vi "Dashboard Main.vi"() -> ()   [LabVIEW 2019]
uses:
  Corsair_V2/Team Code/TurretMode.ctl
  <vilib>/Utility/miscctls.llb/LVRowAndColumnTypeDef.ctl
  <vilib>/event_ctls.llb/eventvkey.ctl
  <vilib>/Rock Robotics/Network Tables/NT Read Boolean.vi
  <vilib>/Rock Robotics/WPI/Dashboard/WPI_DashboardLogging Global.vi
panel:
  in  "Camera Settings Right":T1={"Frame Rate"=30, "Compression"=30, "Size"=1, "DB Camera Config"=FALSE} {"Frame Rate" scale=1.0..30.0; "Compression" scale=100.0..-1.0; "Size" items=["640x480", "320x240", "160x120"]}
  in  "Camera Name Right":string(combo)="No Camera Selection"
  out "Camera Perf":string
  in  "Camera Settings":T1={"Frame Rate"=30, "Compression"=30, "Size"=1, "DB Camera Config"=FALSE} {"Frame Rate" scale=1.0..30.0; "Compression" scale=100.0..-1.0; "Size" items=["640x480", "320x240", "160x120"]}
  in  "TCP":refnum<k5>
  in  "Rec Mode":enum32{"Stop", "Record", "Playback"}(radio)
  out "Robot IP":string
  out "Image Message":string="Timeout in Camera Communications"
  in  "Dashboard Tab":T2(tab)
  in  "Autonomous Selector":u16(ring) items=["3 Ball", "5 Ball"]
  out "Intake jam?":bool
  out "Climber on?":bool
  out "Ball in conveyor?":bool
  out "A valid target?":bool
  out "Right":dbl
  out "Left":dbl
  out "Range?":bool
  out "Mode":T3(ring)=enum."Auto Disabled"
  out "Right Camera Perf":cluster{"Bandwidth (Mbps)":dbl, "FPS":dbl}
  out "Background":bool
  out "Camera Image Right":T4(plugin-control)
  out "BallState":T5(ring)
  out "TurretMode":T6
  out "ClimberState":T7(ring)
  out "RightMotorsTemperature":dbl
  out "LeftMotorsTemperature":dbl
  out "IntakeOutput":dbl
  out "RollerOutput":dbl
  out "TurretEncoder":dbl
  out "Flywheel":dbl
  in  "Select Auto":string(combo)="Select Autonomous ..."
  in  "Test Slider":dbl(slide) scale=0.0..100.0 scale format="%#_3g"
  in  "On/Off":bool caption="Solenoid"
  in  "Test Name":u16(ring) items=["Select the test to run..."]
  in  "Test Tree":string(tree)
  in  "Motor":cluster{"Value":dbl, "Enable":bool} {"Value" scale=-1.0..1.0 scale format="%#_3g"}
  out "Progress":T8 {"Test Progress" scale=0.0..100.0}
  in  "Rev/Fwd":cluster{"Forward":bool, "Reverse":bool}
  in  "Test Ring":u16(ring) items=["Monochrome", "Color"]
  out "Cmd Status":string
  in  "Execute Command":bool
  in  "Command Params":string[][](table)
  in  "Command Selection":i32(listbox)
  in  "CheckList":i32(listbox)
  out "Tree":string(tree)
  out "Camera Image":T4(plugin-control)
  in  "Camera Name":string(combo)="No Camera Selection"
  # "HW"
  # "HW"
  # "Has Limelight"
  # "Turret needs to go to:"
  # "This tab is a great place for autonomous settings and robot-specific values.\nPlace controls and indicators inside this tab and match name to\nDashboard Variables on robot. You can also delete this comment."
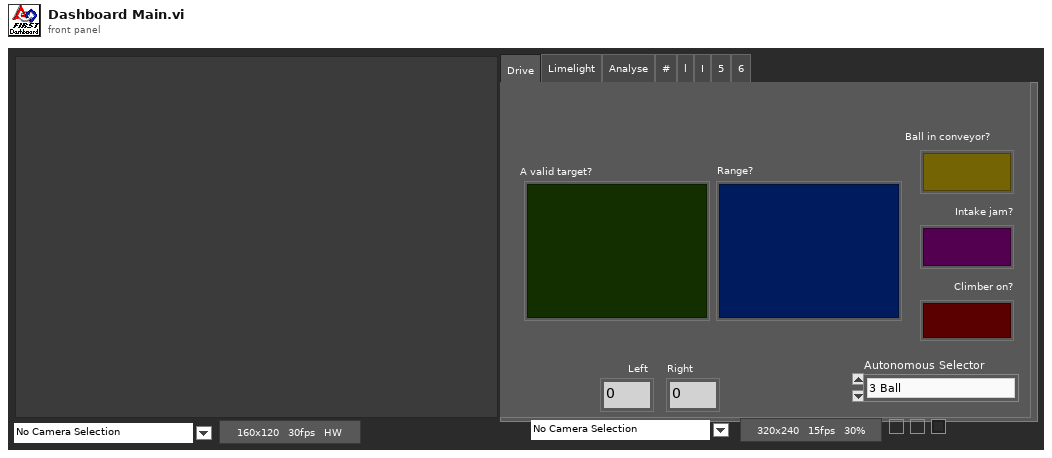
[diagram p1: front panel]
types:
  T1 = cluster{"Frame Rate":i32, "Compression":i32, "Size":u16, "DB Camera Config":bool}
  T2 = enum32{"Drive", "Limelight", "Analyse", "#", "l", "I", "5", "6"}
  T3 = enum8{"Tele-Op Disabled", "Tele-Op Enabled", "Auto Disabled", "Auto Enabled", "Test Disabled", "Test Enabled", "Disconnected", "No Code", "E-Stop"}
  T4 = typedef "IMAQ Image.ctl" = refnum<image>
  T5 = enum16{"Standart", "Get Power Cells", "Balls In", "Prepare Shooter", "Shoot!"}
  T6 = typedef "TurretMode.ctl" = enum16{"Static", "Manual", "Automatic"}
  T7 = enum16{"Standart", "Vibrate *Lenny Face*", "Open da Boi", "Engage on the Bar!", "Pull Our Hope", "Deu por Hoje"}
  T8 = cluster{"Test Progress":u8, "Test Progress Text":string}
  T9 = cluster{"Save Path":path, "Interval (s)":dbl, "Keep":i32}
  T10 = enum32{"Drive", "Camera", "Basic", "Custom", "Test", "Commands", "Checklist", "Variables"}
  T11 = typedef "Image Type" = u32
  T12 = cluster{"IDs":cluster{"RPC field ID":u16, "Unique ID":u16}, "String":string}
  T13 = cluster{"Error Strings":string, "Disable Counts":cluster{u16, u16}, "Rail Faults":cluster{u16, u16, u16}, "Robot IP":string, "DB Mode":u8, "Event Info":cluster{"Name":string, "Type":u8, "Number":u16, "Replay":u8}}
  T14 = cluster{"Storage":cluster{"Disk Free":u64, "RAM Block":u32, "RAM free":u32}, "CPU Utilization":cluster{"CPU % ISR":sgl, "CPU % Time Crit":sgl, "CPU % Timed Str":sgl, "CPU % High":sgl, "CPU % Above":sgl, "CPU % Normal":sgl, "CPU % Low":sgl}, "CAN":cluster{"% Bus Utilization":sgl, "Bus Off Cnt":u32, "TX_FIFO Full Cnt":u32, "Receive Error Cnt":u8, "Transmit Error Cnt":u8}, "HID":cluster{"HID Outputs":u32, "Rumble Low":u16, "Rumble High":u16}[]}
  T15 = cluster{"Status bits":cluster{"Test Mode":bool, "Autonomous":bool, "Enabled":bool, "Code Start":bool, "Brownout":bool, "Reserved 2":bool, "Reserved 3":bool, "E-Stop":bool}, "Code Trace":cluster{"Disabled":bool, "TeleOp":bool, "Auto":bool, "Test":bool}, "Controller Type":enum16{"unknown", "cRIO", "roboRio"}, "Code?":enum16{"unknown", "noCode", "code"}, "Battery V":dbl}
  T16 = cluster{"Control Bits":cluster{"TestMode":bool, "Autonomous":bool, "Enabled":bool, "FMS Present":bool, bool, bool, bool, "E-Stop":bool}, "Team Station ":u8, "Countdown":sgl, "Joystick Values":cluster{"Axes":dbl[], "Buttons":bool[], "POVs":i16[]}[]}
  T17 = cluster{"Camera Image":refnum<vi>, "Dashboard Tab":refnum<vi>, "Background":refnum<vi>, "Rec Mode":refnum<vi>, "Test Slider":refnum<vi>, "On/Off ":refnum<vi>, "Test Ring":refnum<vi>, "Rev/Fwd":refnum<vi>, "Test Name":refnum<vi>, "Motor":refnum<vi>, "Progress":refnum<vi>, "CheckList":refnum<vi>, "Tree":refnum<vi>, "Test Tree":refnum<vi>, "Command Params":refnum<vi>, "Command Selection":refnum<vi>, "Execute Command":refnum<vi>, "Cmd Status":refnum<vi>, "Camera Settings":refnum<vi>, "Camera Name":refnum<vi>, "Camera Perf":refnum<vi>, "Camera Settings Right":refnum<vi>, "Camera Name Right":refnum<vi>, "Camera Image Right":refnum<vi>}
  T18 = cluster{"Global Rectangle":i32[], "Contours":cluster{"Contour Type":u32, "ROI Type":u32, "Points":i32[]}[]}
  T19 = cluster{"Camera Name":string, string, "Saved DB Images Info":cluster{"Save Path":path, "Interval (s)":dbl, "Keep":i32}}
  T20 = cluster{"Camera Name Right":string, string, "Saved DB Images Info":cluster{"Save Path":path, "Interval (s)":dbl, "Keep":i32}}
  T21 = cluster{"Operation":enum16{"Update", "Clear"}, "Color Box":u32}[]
  T22 = typedef "eventvkey.ctl" = enum16{"ASCII", "Enter", "Return", "Shift", "Ctrl", "Alt", "Cmd", "Opt", "Caps", "NumLock", "Clear", "Break", "Up", "Down", "Left", "Right", "Insert", "Delete", "Home", "End", "PageUp", "PageDown", "Escape", "Help", "Pause", "ScrollLock", "F1", "F2", "F3", "F4", "F5", "F6", "F7", "F8", "F9", "F10", "F11", "F12", "F13", "F14", "F15", "F16", "F17", "F18", "F19", "F20", "F21", "F22", "F23", "F24", "Play", "VolumeUp", "VolumeDown", "Mute", "Two Byte Char"}
  T23 = cluster{"Image Size":bool, "Image Type":bool, "Pixel Value":bool, "ROI Information":bool, "Zoom Factor":bool}
  T24 = cluster{"Operation":enum16{"Update", "Clear"}, "Color Box":u32}
  T25 = typedef "LVRowAndColumnTypeDef.ctl" = cluster{"Row":i32, "Column":i32}
  T26 = cluster{"Shift":bool, "Ctrl":bool, "Alt":bool, "Cmd":bool, "Opt":bool}
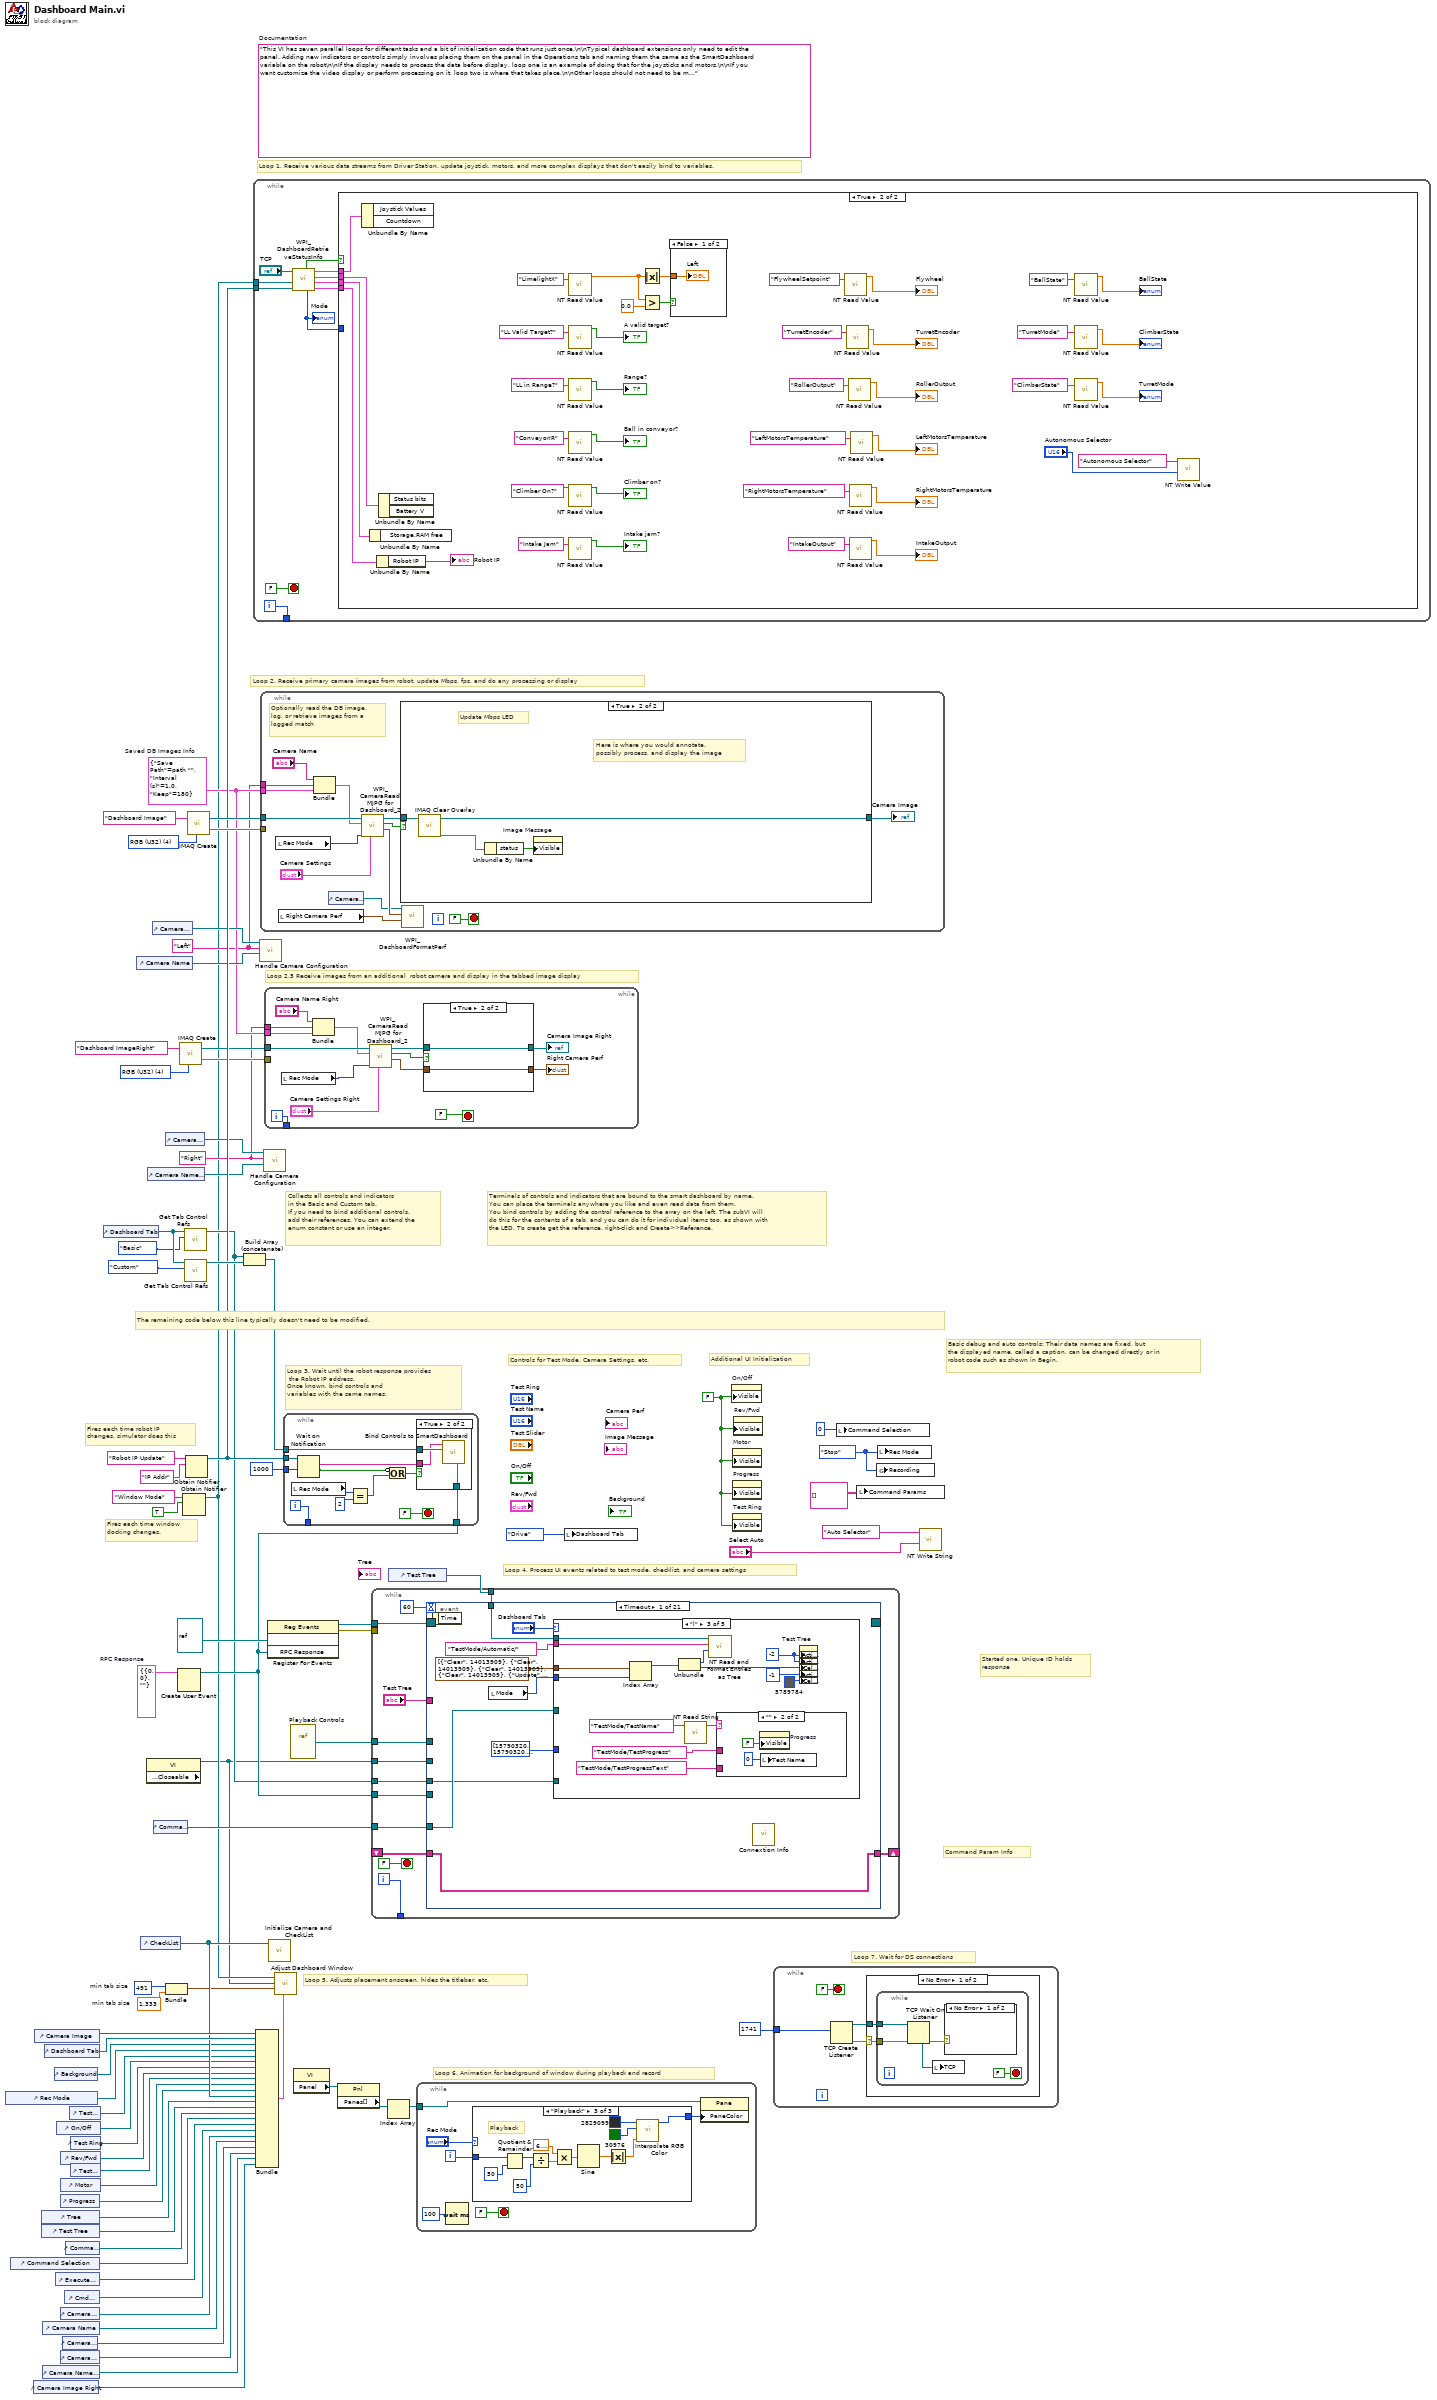
[diagram p0: block diagram]
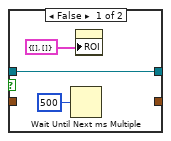
[diagram p2: hidden frame]
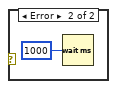
[diagram p3: hidden frame]
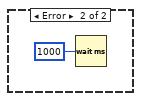
[diagram p4: hidden frame]
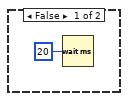
[diagram p5: hidden frame]
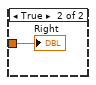
[diagram p6: hidden frame]
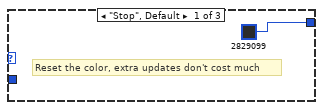
[diagram p7: hidden frame]
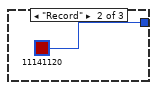
[diagram p8: hidden frame]
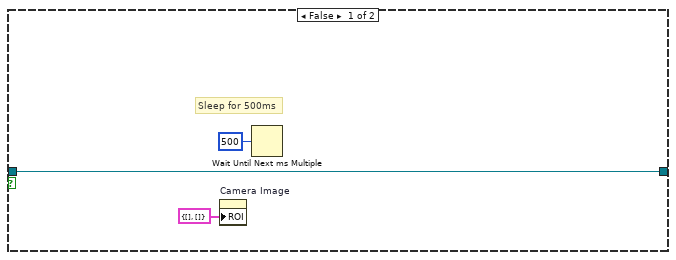
[diagram p10: hidden frame]
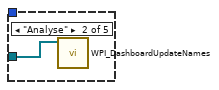
[diagram p12: hidden frame]
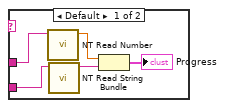
[diagram p13: hidden frame]
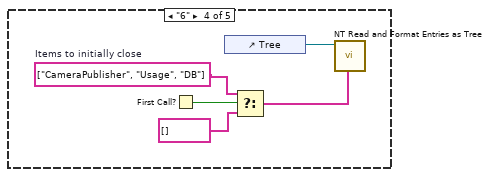
[diagram p14: hidden frame]
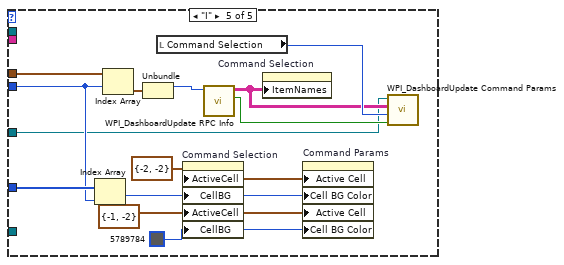
[diagram p15: hidden frame]
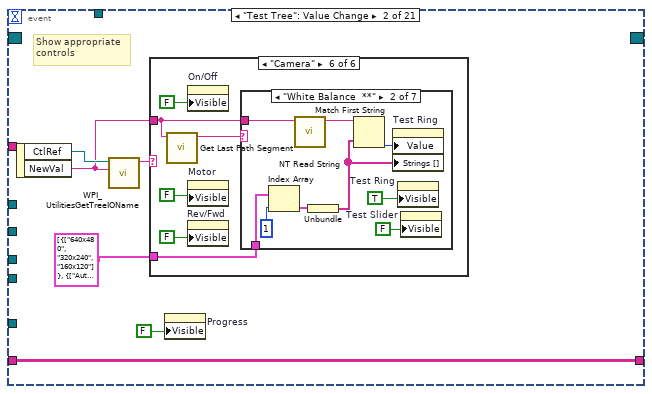
[diagram p16: hidden frame]
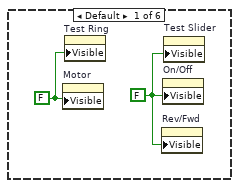
[diagram p17: hidden frame]
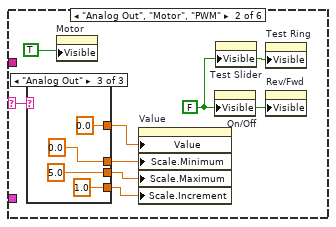
[diagram p18: hidden frame]
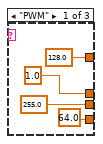
[diagram p19: hidden frame]
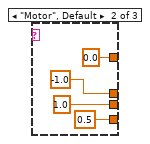
[diagram p20: hidden frame]
diagram:
  w9 = T9 {"Save Path"=path "", "Interval (s)"=1.0, "Keep"=180}  # Saved DB Images Info
  w8 = "Right"
  w7 = "Left"
  w19 = T11 4 items=["Grayscale (U8)", "Grayscale (I16)", "Grayscale (SGL)", "Complex (CSG)", "RGB (U32)", "HSL (U32)", "RGB (U64)"] ("Image Type")
  w35 = T12 {"IDs"={"RPC field ID"=0, "Unique ID"=0}, "String"=""}  # RPC Response
  w53 = 491  # min tab size
  w52 = 1.333  # min tab size
  w59 = enum32{"Stop", "Record", "Playback"}."Stop" ("Rec Mode")
  w41 = FALSE ("Visible")
  (unwired) "This VI has seven parallel loops for different tasks and a bit of initialization code that runs just once.\n\nTypical dashboard extensions only need to edit the panel. Adding new indicators or controls simply involves placing them on the panel in the Operations tab and naming them the same as the SmartDashboard variable on the robot\n\nIf the display needs to process the data before display, loop one is an example of doing that for the joysticks and motors.\n\nIf you want customize the video display or perform processing on it, loop two is where that takes place.\n\nOther loops should not need to be modified. They are pretty standard, and document the task they perform."  # Documentation
  w76 = T11 4 items=["Grayscale (U8)", "Grayscale (I16)", "Grayscale (SGL)", "Complex (CSG)", "RGB (U32)", "HSL (U32)", "RGB (U64)"] ("Image Type")
  # "Loop 2.5 Receive images from an additional  robot camera and display in the tabbed image display"
  # "Command Param Info"
  # "Started one, Unique ID holds\nresponse"
  # "Loop 7. Wait for DS connections"
  # "Basic debug and auto controls: Their data names are fixed, but\nthe displayed name, called a caption, can be changed directly or in\nrobot code such as shown in Begin."
  # "Controls for Test Mode, Camera Settings, etc."
  # "Additional UI Initialization"
  # "Loop 6. Animation for background of window during playback and record"
  # "Fires each time robot IP\nchanges, simulator does this"
  # "Fires each time window\ndocking changes."
  # "Collects all controls and indicators\nin the Basic and Custom tab.\nIf you need to bind additional controls,\nadd their references. You can extend the\nenum constant or use an integer."
  # "The remaining code below this line typically doesn't need to be modified."
  # "Loop 4. Process UI events related to test mode, checklist, and camera settings"
  # "Terminals of controls and indicators that are bound to the smart dashboard by name.\nYou can place the terminals anywhere you like and even read data from them.\nYou bind controls by adding the control reference to the array on the left. The subVI will\ndo this for the contents of a tab, and you can do it for individual items too, as shown with\nthe LED. To create get the reference, right-click and Create>>Reference."
  # "Loop 3. Wait until the robot response provides\n the Robot IP address.\nOnce known, bind controls and\nvariables with the same names."
  # "Loop 5. Adjusts placement onscreen, hides the titlebar, etc."
  # "Loop 1. Receive various data streams from Driver Station, update joystick, motors, and more complex displays that don't easily bind to variables."
  # "Loop 2. Receive primary camera images from robot, update Mbps, fps, and do any processing or display"
  n1 = control-ref of="Rec Mode"() -> (w3:refnum<vi>)
  n2 = control-ref of="Command Selection"() -> (w34:refnum<vi>)
  n3 = control-ref of="Camera Image Right"() -> (w12:refnum<vi>)
  n4 = control-ref of="Camera Image"() -> (w55:refnum<vi>)
  n5 = control-ref of="Tree"() -> (w50:refnum<vi>)
  n6 = control-ref of="Test Tree"() -> (w49:refnum<vi>)
  n7 = control-ref of="Camera Name"() -> (w25:refnum<vi>)
  n8 = control-ref of="Camera Name Right"() -> (w13:refnum<vi>)
  n9 = control-ref of="Dashboard Tab"() -> (w54:refnum<vi>)
  n10 = control-ref of="Background"() -> (w2:refnum<vi>)
  n11 = control-ref of="Execute Command"() -> (w36:refnum<vi>)
  n12 = control-ref of="On/Off"() -> (w45:refnum<vi>)
  n13 = control-ref of="Progress"() -> (w42:refnum<vi>)
  n14 = control-ref of="Camera Settings"() -> (w26:refnum<vi>)
  n15 = control-ref of="Camera Settings Right"() -> (w14:refnum<vi>)
  n16 = control-ref of="Rev/Fwd"() -> (w43:refnum<vi>)
  n17 = control-ref of="Motor"() -> (w47:refnum<vi>)
  n18 = control-ref of="Camera Perf"() -> (w24:refnum<vi>)
  n19 = control-ref of="Cmd Status"() -> (w30:refnum<vi>)
  n20 = control-ref of="Command Params"() -> (w37:refnum<vi>)
  n21 = control-ref of="Test Slider"() -> (w46:refnum<vi>)
  n22 = control-ref of="Test Ring"() -> (w44:refnum<vi>)
  n23 = control-ref of="Test Name"() -> (w48:refnum<vi>)
  n24 = control-ref of="Dashboard Tab"() -> (w58:refnum<vi>)
  n25 = control-ref of="Camera Name"() -> (w27:refnum<vi>)
  n26 = control-ref of="CheckList"() -> (w51:refnum<vi>)
  n27 = property class="VI" props=["Front Panel.Closeable"]() -> (reference out=w4:refnum<vi>)  [unwired: 2 in, 2 out]
  n28 = control-ref of="Camera Name Right"() -> (w15:refnum<vi>)
  n29 = control-ref of="Camera Settings"() -> (w28:refnum<vi>)
  n30 = control-ref of="Command Params"() -> (w29:refnum<vi>)
  n31 = control-ref of="Camera Settings Right"() -> (w16:refnum<vi>)
  n32 = Bundle("min tab size"=w53, "min tab size"=w52) -> (w6:cluster{"min tab size":i32, "min tab size":dbl})  [unwired: 1 in]
  n33 = Create User Event(user event datatype=w35) -> (user event=w31:refnum<user-event>)  [unwired: 1 in, 1 out]
  n34 = call "IMAQ Create"("Image Name"="Dashboard ImageRight", "Image Type"=w19) -> ("New Image"=w18:T4, "error out"=w17:errorcluster)  [unwired: 2 in, 1 out]
  n35 = Obtain Notifier(name (unnamed)="Window Mode", notification data type=TRUE) -> (notifier out=w5:refnum<notifier>)  [unwired: 2 in, 2 out]
  n36 = call <vilib>:"Get Tab Control Refs.vi"("Page Index"=T10."Basic" ("Dashboard Tab"), "TabControl in"=w58) -> ("ControlsOnPage"=w23:refnum<vi>[])  [unwired: 9 in]
  n37 = call <vilib>:"Get Tab Control Refs.vi"("Page Index"=T10."Custom" ("Dashboard Tab"), "TabControl in"=w58) -> ("ControlsOnPage"=w57:refnum<vi>[])  [unwired: 9 in]
  n38 = Obtain Notifier(name (unnamed)="Robot IP Update", notification data type="IP Addr" ("name (unnamed)")) -> (notifier out=w40:refnum<notifier>)  [unwired: 2 in, 2 out]
  n39 = call "IMAQ Create"("Image Name"="Dashboard Image", "Image Type"=w76) -> ("New Image"=w74:T4, "error out"=w73:errorcluster)  [unwired: 2 in, 1 out]
  n40 = Build Array (concatenate)(w23, w57) -> (w56:refnum<vi>[])
  n41 = while {
    tunnel: [w86] -> _
    tunnel: w40 -> [w80]
    tunnel: w5 -> [w77]
    i -> [w86]
    stop <- FALSE stop-if-true
    n42 = call <vilib>:"WPI_DashboardRetrieveStatusInfo.vi"("Binding Refnum"=w80, "Window Mode Notifier"=w77, "TCP Cnx"="TCP") -> ("Power and Errors"=w81:T13, "Robot Metrics"=w84:T14, "Status Info"=w85:T15, "Control Info"=w82:T16, "Robot Mode"=w79:T3, "Process?"=w83:bool)  [unwired: 3 in]
    "Mode" <- w79
    n43 = case shown="True" w83 {
      tunnel: w85 -> [_ w128]
      tunnel: w84 -> [_ w127]
      tunnel: w82 -> [_ w126]
      tunnel: w81 -> [_ w125]
      tunnel: w79 -> [_ _]
      frame False {
        n44 = Wait (ms)(milliseconds to wait=u32 20) -> ()  [unwired: 1 out]
      }
      frame True {
        n45 = Unbundle By Name(w126) -> ()  [unwired: 2 out]
        n46 = Unbundle By Name(w127) -> ()  [unwired: 1 out]
        n47 = Unbundle By Name(w125) -> ("Robot IP"=→"Robot IP":string)
        n48 = Unbundle By Name(w128) -> ()  [unwired: 2 out]
        n49 = call-poly <vilib>:"NT Read Value.vi"("Name"="LimelightX") -> ("Numeric"=w120:dbl)  [unwired: 9 in, 1 out]
        n50 = call-poly <vilib>:"NT Read Value.vi"("Name"="LL Valid Target?") -> ("Boolean"=→"A valid target?":bool)  [unwired: 9 in, 1 out]
        n51 = call-poly <vilib>:"NT Read Value.vi"("Name"="LL in Range?") -> ("Boolean"=→"Range?":bool)  [unwired: 9 in, 1 out]
        n52 = call-poly <vilib>:"NT Read Value.vi"("Name"="ConveyorIR") -> ("Boolean"=→"Ball in conveyor?":bool)  [unwired: 9 in, 1 out]
        n53 = call-poly <vilib>:"NT Read Value.vi"("Name"="Climber On?") -> ("Boolean"=→"Climber on?":bool)  [unwired: 9 in, 1 out]
        n54 = call-poly <vilib>:"NT Read Value.vi"("Name"="Intake Jam") -> ("Boolean"=→"Intake jam?":bool)  [unwired: 9 in, 1 out]
        n55 = Absolute Value(x=w120) -> (abs(x)=w119:dbl)
        n56 = Greater?(x=w120, y=0.0) -> (0:w121:bool)
        n57 = case shown="False" w121 {
          tunnel: w119 -> [w129 w130]
          frame False {
            "Left" <- w129
          }
          frame True {
            "Right" <- w130
          }
        }
        n58 = call-poly <vilib>:"NT Read Value.vi"("Name"="FlywheelSetpoint") -> ("Numeric"=→"Flywheel":dbl)  [unwired: 9 in, 1 out]
        n59 = call-poly <vilib>:"NT Read Value.vi"("Name"="TurretEncoder") -> ("Numeric"=→"TurretEncoder":dbl)  [unwired: 9 in, 1 out]
        n60 = call-poly <vilib>:"NT Read Value.vi"("Name"="RollerOutput") -> ("Numeric"=→"RollerOutput":dbl)  [unwired: 9 in, 1 out]
        n61 = call-poly <vilib>:"NT Read Value.vi"("Name"="RightMotorsTemperature") -> ("Numeric"=→"RightMotorsTemperature":dbl)  [unwired: 9 in, 1 out]
        n62 = call-poly <vilib>:"NT Read Value.vi"("Name"="IntakeOutput") -> ("Numeric"=→"IntakeOutput":dbl)  [unwired: 9 in, 1 out]
        n63 = call-poly <vilib>:"NT Read Value.vi"("Name"="LeftMotorsTemperature") -> ("Numeric"=→"LeftMotorsTemperature":dbl)  [unwired: 9 in, 1 out]
        n64 = call-poly <vilib>:"NT Read Value.vi"("Name"="BallState") -> ("Numeric"=→"BallState":dbl)  [unwired: 9 in, 1 out]
        n65 = call-poly <vilib>:"NT Read Value.vi"("Name"="TurretMode") -> ("Numeric"=→"ClimberState":dbl)  [unwired: 9 in, 1 out]
        n66 = call-poly <vilib>:"NT Read Value.vi"("Name"="ClimberState") -> ("Numeric"=→"TurretMode":dbl)  [unwired: 9 in, 1 out]
        n67 = call-poly <vilib>:"NT Write Value.vi"("Numeric"="Autonomous Selector", "Name"="Autonomous Selector") -> ()  [unwired: 9 in, 1 out]
      }
    }
  }
  n68 = Bundle("Camera Image"=w55, "Dashboard Tab"=w54, "Background"=w2, "Rec Mode"=w3, "Test Slider"=w46, "On/Off"=w45, "Test Ring"=w44, "Rev/Fwd"=w43, "Test Name"=w48, "Motor"=w47, "Progress"=w42, "CheckList"=w51, "Tree"=w50, "Test Tree"=w49, "Command Params"=w37, "Command Selection"=w34, "Execute Command"=w36, "Cmd Status"=w30, "Camera Settings"=w26, "Camera Name"=w25, "Camera Perf"=w24, "Camera Settings Right"=w14, "Camera Name Right"=w13, "Camera Image Right"=w12) -> (w1:T17)  [unwired: 1 in]
  n69 = call "Handle Camera Configuration.vi"("CameraNameRef"=w27, "Display Name"=w7, "ClusterRef"=w28) -> ()  [unwired: 9 in]
  n70 = while {
    tunnel: w74 -> [w143]
    tunnel: w73 -> [_]
    tunnel: w9 -> [w137]
    tunnel: w7 -> [w134]
    stop <- FALSE stop-if-true
    # "Optionally read the DB image,\nlog, or retrieve images from a\nlogged match"
    n71 = local read "Rec Mode"() -> (w140:enum32{"Stop", "Record", "Playback"})
    n72 = local read "Right Camera Perf"() -> (w132:cluster{"Bandwidth (Mbps)":dbl, "FPS":dbl})
    n73 = Bundle("Camera Name"="Camera Name", w134, "Saved DB Images Info"=w137) -> (w136:T19)  [unwired: 1 in]
    n74 = control-ref of="Camera Perf"() -> (w131:refnum<vi>)
    n75 = call <vilib>:"WPI_CameraRead MJPG for Dashboard_2.vi"("Camera Settings"="Camera Settings", "Rec Mode"=w140, "Capture Info"=w136, "Image in"=w143) -> ("perf info"=w133:cluster{"Bandwidth (Mbps)":dbl, "fps":dbl}, "Active"=w141:bool, "Image\\ out"=w142:T4)  [unwired: 5 in]
    n76 = case shown="True" w141 {
      tunnel: w142 -> [w146 w149]
      tunnel: [w146 w148] -> w138
      frame False {
        # "Sleep for 500ms"
        n77 = property on="Camera Image" class="ImageControl"("ROI"=T18 {"Global Rectangle"=[], "Contours"=[]}) -> ()  [unwired: 2 in, 2 out]
        n78 = Wait Until Next ms Multiple(millisecond multiple=u32 500) -> ()  [unwired: 1 out]
      }
      frame True {
        # "Here is where you would annotate,\npossibly process, and display the image"
        # "Update Mbps LED"
        n79 = call "IMAQ Clear Overlay"("Image"=w149) -> ("error out"=w150:errorcluster, "Image Out"=w148:T4)  [unwired: 2 in, 7 out]
        n80 = Unbundle By Name(w150) -> ("status"=w151:bool)
        n81 = property on="Image Message" class="Str"("Visible"=w151) -> ()  [unwired: 2 in, 2 out]
      }
    }
    "Camera Image" <- w138
    n82 = call <vilib>:"WPI_DashboardFormatPerf.vi"("Right Camera Perf"=w132, "Performance"=w133, "String in"=w131) -> ()  [unwired: 9 in]
  }
  n83 = call "Handle Camera Configuration.vi"("CameraNameRef"=w15, "Display Name"=w8, "ClusterRef"=w16) -> ()  [unwired: 9 in]
  n84 = while {
    tunnel: w18 -> [w165]
    tunnel: w17 -> [_]
    tunnel: [w160] -> _
    tunnel: w9 -> [w157]
    tunnel: w8 -> [w154]
    i -> [w160]
    stop <- FALSE stop-if-true
    n85 = local read "Rec Mode"() -> (w164:enum32{"Stop", "Record", "Playback"})
    n86 = Bundle("Camera Name Right"="Camera Name Right", w154, "Saved DB Images Info"=w157) -> (w156:T20)  [unwired: 1 in]
    n87 = call <vilib>:"WPI_CameraRead MJPG for Dashboard_2.vi"("Camera Settings"="Camera Settings Right", "Rec Mode"=w164, "Capture Info"=w156, "Image in"=w165) -> ("perf info"=w152:cluster{"Bandwidth (Mbps)":dbl, "fps":dbl}, "Active"=w159:bool, "Image\\ out"=w162:T4)  [unwired: 5 in]
    n88 = case shown="True" w159 {
      tunnel: w162 -> [w167 w170]
      tunnel: [w167 w170] -> w158
      tunnel: [_ w169] -> w153
      tunnel: w152 -> [_ w169]
      frame False {
        n89 = Wait Until Next ms Multiple(millisecond multiple=u32 500) -> ()  [unwired: 1 out]
        n90 = property on="Camera Image Right" class="ImageControl"("ROI"=T18 {"Global Rectangle"=[], "Contours"=[]}) -> ()  [unwired: 2 in, 2 out]
      }
      frame True {
      }
    }
    "Camera Image Right" <- w158
    "Right Camera Perf" <- w153
  }
  n91 = register-events(refnum<vi> refnum, w31) -> (reference out=w63:refnum<event-registration>, error out=w62:errorcluster)  [unwired: 2 in]
  n92 = call "Initialize Camera and CheckList.vi"("ListBox in"=w51) -> ()  [unwired: 11 in]
  n93 = call "Adjust Dashboard Window.vi"("Sizing Refnums"=w1, "Size Constraints"=w6, "VI"=w4, "WIn Mode"=w5) -> ()  [unwired: 8 in]
  n94 = while {
    tunnel: w56 -> [w182]
    tunnel: w40 -> [w180]
    tunnel: [w178] -> _
    tunnel: u32 1000 ("milliseconds to wait") -> [w177]
    tunnel: w31 -> [w171]
    i -> [w178]
    stop <- FALSE stop-if-true
    n95 = local read "Rec Mode"() -> (w173:enum32{"Stop", "Record", "Playback"})
    n96 = Wait on Notification(notifier=w180, timeout in ms (-1)=w177) -> (notification=w179:string, timed out?=w175:bool)  [unwired: 2 in, 2 out]
    n97 = Equal?(x=w173, y=u16 2 ("Rec Mode")) -> (x = y?=w174:bool)
    n98 = Compound Arithmetic op=OR(invert w175, w174) -> (w176:bool)
    n99 = case shown="True" w176 {
      tunnel: w182 -> [_ w185]
      tunnel: w179 -> [_ w184]
      tunnel: w171 -> [_ w183]
      frame False {
      }
      frame True {
        n100 = call <vilib>:"Bind Controls to SmartDashboard.vi"("RPC ref"=w183, "Bound Control Refs"=w185, "Server IP Address"=w184) -> ()  [unwired: 9 in]
      }
    }
  }
  n101 = vi-ref "Playback Controls.vi"() -> (w64:refnum<vi>)
  n102 = property class="VI"() -> ("Panel"=w66:refnum<vi>)  [unwired: 2 in, 2 out]
  n103 = property class="Pnl"(reference=w66) -> ("Panes[]"=w67:refnum<vi>[])  [unwired: 1 in, 2 out]
  n104 = Index Array(array=w67) -> (element=w65:refnum<vi>)  [unwired: 1 in]
  n105 = control-ref of="Test Tree"() -> (w68:refnum<vi>)
  n106 = while {
    tunnel: [w195] -> _
    tunnel: w68 -> [w194]
    tunnel: w64 -> [w193]
    tunnel: w63 -> [w192]
    tunnel: w62 -> [_]
    tunnel: w4 -> [w191]
    tunnel: w31 -> [w190]
    tunnel: w29 -> [w189]
    shift-right: [w188] -> _
    shift-left: _ -> [w187]
    tunnel: w23 -> [w186]
    i -> [w195]
    stop <- FALSE stop-if-true
    n107 = event shown="[0] Timeout" {
      selector: w192 -> [_ _ _ _ _ _ _ _ _ _ _ _ _ _ _ _ _ _ _ _ _]
      dyn-events: [_ _ _ _ _ _ _ _ _ _ _ _ _ _ _ _ w454 _ _ _ _] -> _
      timeout: u32 60 ("milliseconds to wait") -> [_ _ _ _ _ _ _ _ _ _ _ _ _ _ _ _ _ _ _ _ _]
      tunnel: w194 -> [w207 _ _ _ _ _ _ _ _ _ _ _ _ _ _ _ _ _ _ _ _]
      tunnel: "Test Tree" -> [_ _ _ _ _ _ _ _ _ _ _ w421 w429 w431 w435 w443 _ _ _ _ _]
      tunnel: w193 -> [_ _ _ _ _ _ _ _ _ _ _ _ _ _ _ _ w456 _ w474 _ _]
      tunnel: w191 -> [_ _ _ _ _ _ _ _ _ _ _ _ _ _ _ _ w452 _ _ _ _]
      tunnel: w190 -> [_ _ _ _ _ _ _ _ _ _ _ _ _ _ _ _ w450 _ _ _ _]
      tunnel: w189 -> [w203 _ _ _ _ _ w372 _ _ _ _ _ _ _ _ _ _ _ _ _ _]
      tunnel: [w202 w249 w351 w356 w365 w369 w370 w379 w389 w396 w408 w420 w427 w430 w434 w442 w449 w469 w471 w475 w488] -> w188
      tunnel: w187 -> [w202 w249 w351 w356 w365 w369 w370 _ _ w396 w408 w420 w427 w430 w434 w442 w449 w469 w471 w475 w488]
      tunnel: w186 -> [w200 _ _ _ _ _ _ _ _ _ _ _ _ _ _ _ _ _ _ _ _]
      event Timeout {
        n108 = event-data() -> ()  [unwired: 1 in, 1 out]
        n109 = local read "Mode"() -> (w205:T3)
        n110 = case shown="\"l\"" "Dashboard Tab" {
          tunnel: w207 -> [_ _ w222 _ _]
          tunnel: "TestMode/Automatic/" ("Name Pattern") -> [_ _ w221 _ _]
          tunnel: T21 [{"Operation"=enum."Clear", "Color Box"=14013909}, {"Operation"=enum."Clear", "Color Box"=14013909}, {"Operation"=enum."Clear", "Color Box"=14013909}, {"Operation"=enum."Clear", "Color Box"=14013909}, {"Operation"=enum."Update", "Color Box"=14013909}, {"Operation"=enum."Update", "Color Box"=16777215}, {"Operation"=enum."Clear", "Color Box"=14013909}, {"Operation"=enum."Clear", "Color Box"=14013909}, {"Operation"=enum."Clear", "Color Box"=14013909}] -> [_ _ w214 _ w242]
          tunnel: w205 -> [_ _ w213 _ w241]
          tunnel: u32[] [15790320, 15790320, 15790320, 15790320, 16777215, 16777215, 15790320, 15790320, 15790320] -> [_ _ _ _ w247]
          tunnel: w203 -> [_ _ _ _ w235]
          tunnel: w200 -> [_ w208 _ _ _]
          frame "Limelight", Default {
          }
          frame "Analyse" {
            n111 = call <vilib>:"WPI_DashboardUpdateNames.vi"("Controls on Tab"=w208) -> ()  [unwired: 11 in]
          }
          frame "l" {
            w220 = -2 ("Active Item:Row Number")
            n112 = Index Array(array=w214, index=w213) -> (element=w215:T24)
            n113 = Unbundle(w215) -> ("Operation"=w216:enum16{"Update", "Clear"}, "Color Box"=w217:u32)
            n114 = call <vilib>:"NT Read String.vi"("Name"="TestMode/TestName") -> ("String"=w211:string)  [unwired: 9 in, 1 out]
            n115 = call <vilib>:"NT Read and Format Entries as Tree.vi"("Operation"=w216, "Name Pattern"=w221, "Tree Refnum"=w222) -> ()  [unwired: 7 in, 2 out]
            n116 = case shown="\"\"" w211 {
              tunnel: "TestMode/TestProgress" ("Name") -> [w224 _]
              tunnel: "TestMode/TestProgressText" ("Name") -> [w223 _]
              frame Default {
                n117 = call <vilib>:"NT Read Number.vi"("Name"=w224) -> ("Numeric"=w225:dbl)  [unwired: 9 in, 1 out]
                n118 = call <vilib>:"NT Read String.vi"("Name"=w223) -> ("String"=w226:string)  [unwired: 9 in, 1 out]
                n119 = Bundle("Numeric"=w225, "String"=w226) -> (→"Progress":cluster{"Numeric":dbl, "String":string})  [unwired: 1 in]
              }
              frame "" {
                n120 = property on="Progress" class="Clust (strict)"("Visible"=FALSE) -> ()  [unwired: 2 in, 2 out]
                n121 = local write "Test Name"(u16 0) -> ()
              }
            }
            n122 = property on="Test Tree" class="Tree (strict)"("Active Item Row Number"=w220, "ActiveColNum"=w220, "CellBG"=w217, "Active Item Row Number"=-1 ("Active Item:Row Number"), "CellBG"=u32 5789784 ("Color Box")) -> ()  [unwired: 2 in, 2 out]
          }
          frame "6" {
            w232 = string[] ["CameraPublisher", "Usage", "DB"]  # Items to initially close
            n123 = First Call?() -> (First Call?: T/F=w233:bool)
            n124 = control-ref of="Tree"() -> (w234:refnum<vi>)
            n125 = Select(t=w232, s=w233, f=string[] []) -> (s? t:f=w230:string[])
            n126 = call <vilib>:"NT Read and Format Entries as Tree.vi"("Tags to  Close"=w230, "Tree Refnum"=w234) -> ()  [unwired: 8 in, 2 out]
          }
          frame "I" {
            w243 = u32 5789784 ("Color Box")
            w244 = T25 {"Row"=-1, "Column"=-2} ("Active Cell:Active Cell")
            w246 = T25 {"Row"=-2, "Column"=-2} ("Active Cell:Active Cell")
            n127 = Index Array(array=w247, index=w241) -> (element=w245:u32)
            n128 = Index Array(array=w242, index=w241) -> (element=w240:T24)
            n129 = Unbundle(w240) -> ("Operation"=w239:enum16{"Update", "Clear"})  [unwired: 1 out]
            n130 = local read "Command Selection"() -> (w238:i32)
            n131 = property on="Command Selection" class="MCListbox (strict)"("ActiveCell"=w246, "CellBG"=w245, "ActiveCell"=w244, "CellBG"=w243) -> ()  [unwired: 2 in, 2 out]
            n132 = call <vilib>:"WPI_DashboardUpdate RPC Info.vi"("Operation"=w239) -> ("update"=w237:bool, "commands"=w236:string[][])  [unwired: 9 in]
            n133 = property on="Command Selection" class="MCListbox (strict)"("ItemNames"=w236) -> ()  [unwired: 2 in, 2 out]
            n134 = property on="Command Params" class="Tbl (strict)"("Active Cell"=w246, "Cell BG Color"=w245, "Active Cell"=w244, "Cell BG Color"=w243) -> ()  [unwired: 2 in, 2 out]
            n135 = call <vilib>:"WPI_DashboardUpdate Command Params.vi"("Update"=w237, "NewVal"=w238, "Commands"=w236, "Param Tbl"=w235) -> ()  [unwired: 7 in, 1 out]
          }
        }
        n136 = call <vilib>:"Connextion Info.vi"() -> ()  [unwired: 10 in, 2 out]
      }
      event "Test Tree": Value Change {
        # "Show appropriate\ncontrols"
        n137 = event-data() -> ("CtlRef"=w252:refnum<vi>, "NewVal"=w250:string)  [unwired: 1 in]
        n138 = call <vilib>:"WPI_UtilitiesGetTreeIOName.vi"("NewVal"=w250, "TreeControl in"=w252) -> ("I/O Name"=w253:string)  [unwired: 9 in]
        n139 = case shown="\"Camera\"" w253 {
          selector: w253 -> [_ w260 _ w282 w291 _]
          tunnel: w250 -> [_ _ w279 w281 _ w298]
          tunnel: cluster{string[]}[] [{["640x480", "320x240", "160x120"]}, {["Auto", "Fixed indoor", "Fixed outdoor 1", "Fixed outdoor 2", "Fixed fluorescent 1", "Fixed fluorescent 2", "Hold current"]}, {["Auto", "Flicker-free 50 Hz", "Flicker-free 60 Hz", "Hold current"]}, {["None", "Prioritize frame rate", "Prioritize image quality"]}, {["Monochrome", "Color"]}] -> [_ _ _ _ _ w297]
          frame Default {
            w255 = FALSE ("Visible")
            w254 = FALSE ("Visible")
            n140 = property on="Motor" class="Clust (strict)"("Visible"=w254) -> ()  [unwired: 2 in, 2 out]
            n141 = property on="Test Ring" class="Ring (strict)"("Visible"=w254) -> ()  [unwired: 2 in, 2 out]
            n142 = property on="Rev/Fwd" class="Clust (strict)"("Visible"=w255) -> ()  [unwired: 2 in, 2 out]
            n143 = property on="On/Off" class="Bool (strict)"("Visible"=w255) -> ()  [unwired: 2 in, 2 out]
            n144 = property on="Test Slider" class="Slide (strict)"("Visible"=w255) -> ()  [unwired: 2 in, 2 out]
          }
          frame "Analog Out", "Motor", "PWM" {
            w261 = FALSE ("Visible")
            n145 = case shown="\"Analog Out\"" w260 {
              tunnel: [1.0 ("Value") -1.0 ("Value") 0.0 ("Value")] -> w259
              tunnel: [255.0 ("Value") 1.0 ("Value") 5.0 ("Value")] -> w258
              tunnel: [128.0 ("Value") 0.0 ("Value") 0.0 ("Value")] -> w257
              tunnel: [64.0 ("Value") 0.5 ("Value") 1.0 ("Value")] -> w256
              frame "PWM" {
              }
              frame "Motor", Default {
              }
              frame "Analog Out" {
              }
            }
            n146 = property on="Motor" class="Clust (strict)"("Visible"=TRUE) -> ()  [unwired: 2 in, 2 out]
            n147 = property on="Value" class="Slide (strict)"("Value"=w257, "Scale.Minimum"=w259, "Scale.Maximum"=w258, "Scale.Increment"=w256) -> ()  [unwired: 2 in, 2 out]
            n148 = property on="On/Off" class="Bool (strict)"("Visible"=w261) -> ()  [unwired: 2 in, 2 out]
            n149 = property on="Test Slider" class="Slide (strict)"("Visible"=w261) -> ()  [unwired: 2 in, 2 out]
            n150 = property on="Test Ring" class="Ring (strict)"("Visible"=w261) -> ()  [unwired: 2 in, 2 out]
            n151 = property on="Rev/Fwd" class="Clust (strict)"("Visible"=w261) -> ()  [unwired: 2 in, 2 out]
          }
          frame "Servo" {
            w277 = FALSE ("Visible")
            n152 = call <vilib>:"NT Read Number.vi"("Name"=w279) -> ("Numeric"=w278:dbl)  [unwired: 9 in, 1 out]
            n153 = property on="Test Slider" class="Slide (strict)"("Visible"=TRUE, "Scale.Maximum"=170.0 ("Scale.Range:Maximum")) -> ()  [unwired: 2 in, 2 out]
            n154 = local write "Test Slider"(w278) -> ()
            n155 = property on="Motor" class="Clust (strict)"("Visible"=w277) -> ()  [unwired: 2 in, 2 out]
            n156 = property on="Rev/Fwd" class="Clust (strict)"("Visible"=w277) -> ()  [unwired: 2 in, 2 out]
            n157 = property on="On/Off" class="Bool (strict)"("Visible"=w277) -> ()  [unwired: 2 in, 2 out]
            n158 = property on="Test Ring" class="Ring (strict)"("Visible"=w277) -> ()  [unwired: 2 in, 2 out]
          }
          frame "Relay", "Solenoid" {
            w280 = FALSE ("Visible")
            n159 = property on="Motor" class="Clust (strict)"("Visible"=w280) -> ()  [unwired: 2 in, 2 out]
            n160 = property on="Test Slider" class="Slide (strict)"("Visible"=w280) -> ()  [unwired: 2 in, 2 out]
            n161 = Search and Replace String(input string=w281, search string="/Value  **", replace string="/Direction") -> (result string=w287:string)  [unwired: 5 in, 3 out]
            n162 = property on="Test Ring" class="Ring (strict)"("Visible"=w280) -> ()  [unwired: 2 in, 2 out]
            n163 = call <vilib>:"NT Read String.vi"("Name"=w287) -> ("String"=w285:string)  [unwired: 9 in, 1 out]
            n164 = Equal?(x="Both directions", y=w285) -> (x = y?=w283:bool)
            n165 = Not(x=w283) -> (.not. x?=w284:bool)
            n166 = property on="Rev/Fwd" class="Clust (strict)"("Visible"=w283) -> ()  [unwired: 2 in, 2 out]
            n167 = property on="On/Off" class="Bool (strict)"("Visible"=w284, "Caption.Text"=w282) -> ()  [unwired: 2 in, 2 out]
          }
          frame "Compressor", "Digital Out" {
            w290 = FALSE ("Visible")
            # "Get direction and finish"
            n168 = property on="Motor" class="Clust (strict)"("Visible"=w290) -> ()  [unwired: 2 in, 2 out]
            n169 = property on="Test Slider" class="Slide (strict)"("Visible"=w290) -> ()  [unwired: 2 in, 2 out]
            n170 = property on="Test Ring" class="Ring (strict)"("Visible"=w290) -> ()  [unwired: 2 in, 2 out]
            n171 = property on="On/Off" class="Bool (strict)"("Visible"=TRUE, "Caption.Text"=w291) -> ()  [unwired: 2 in, 2 out]
            n172 = property on="Rev/Fwd" class="Clust (strict)"("Visible"=FALSE) -> ()  [unwired: 2 in, 2 out]
          }
          frame "Camera" {
            n173 = call <vilib>:"Get Last Path Segment.vi"("String in"=w298) -> ("String out"=w299:string)  [unwired: 10 in]
            n174 = property on="On/Off" class="Bool (strict)"("Visible"=FALSE) -> ()  [unwired: 2 in, 2 out]
            n175 = property on="Motor" class="Clust (strict)"("Visible"=FALSE) -> ()  [unwired: 2 in, 2 out]
            n176 = property on="Rev/Fwd" class="Clust (strict)"("Visible"=FALSE) -> ()  [unwired: 2 in, 2 out]
            n177 = case shown="\"White Balance  **\"" w299 {
              tunnel: w298 -> [w305 w314 w323 w332 w341 _ w347]
              tunnel: w297 -> [w303 w311 w320 w329 w338 _ _]
              frame "Size  **" {
                n178 = Index Array(array=w303) -> (element=w302:cluster{string[]})  [unwired: 1 in]
                n179 = call <vilib>:"NT Read String.vi"("Name"=w305) -> ("String"=w304:string)  [unwired: 9 in, 1 out]
                n180 = Unbundle(w302) -> (w300:string[])
                n181 = Match First String(2:w300, 3:w304) -> (0:w301:i32)  [unwired: 1 out]
                n182 = property on="Test Ring" class="Ring (strict)"("Value"=w301, "Strings []"=w300) -> ()  [unwired: 2 in, 2 out]
                n183 = property on="Test Ring" class="Ring (strict)"("Visible"=TRUE) -> ()  [unwired: 2 in, 2 out]
                n184 = property on="Test Slider" class="Slide (strict)"("Visible"=FALSE) -> ()  [unwired: 2 in, 2 out]
              }
              frame "White Balance  **" {
                n185 = Index Array(array=w311, index=1) -> (element=w312:cluster{string[]})
                n186 = call <vilib>:"NT Read String.vi"("Name"=w314) -> ("String"=w313:string)  [unwired: 9 in, 1 out]
                n187 = Unbundle(w312) -> (w309:string[])
                n188 = Match First String(2:w309, 3:w313) -> (0:w308:i32)  [unwired: 1 out]
                n189 = property on="Test Ring" class="Ring (strict)"("Value"=w308, "Strings []"=w309) -> ()  [unwired: 2 in, 2 out]
                n190 = property on="Test Ring" class="Ring (strict)"("Visible"=TRUE) -> ()  [unwired: 2 in, 2 out]
                n191 = property on="Test Slider" class="Slide (strict)"("Visible"=FALSE) -> ()  [unwired: 2 in, 2 out]
              }
              frame "Exposure  **" {
                n192 = Index Array(array=w320, index=2) -> (element=w321:cluster{string[]})
                n193 = call <vilib>:"NT Read String.vi"("Name"=w323) -> ("String"=w322:string)  [unwired: 9 in, 1 out]
                n194 = Unbundle(w321) -> (w317:string[])
                n195 = Match First String(2:w317, 3:w322) -> (0:w318:i32)  [unwired: 1 out]
                n196 = property on="Test Ring" class="Ring (strict)"("Value"=w318, "Strings []"=w317) -> ()  [unwired: 2 in, 2 out]
                n197 = property on="Test Ring" class="Ring (strict)"("Visible"=TRUE) -> ()  [unwired: 2 in, 2 out]
                n198 = property on="Test Slider" class="Slide (strict)"("Visible"=FALSE) -> ()  [unwired: 2 in, 2 out]
              }
              frame "Exposure Priority  **" {
                n199 = Index Array(array=w329, index=3) -> (element=w330:cluster{string[]})
                n200 = call <vilib>:"NT Read String.vi"("Name"=w332) -> ("String"=w331:string)  [unwired: 9 in, 1 out]
                n201 = Unbundle(w330) -> (w326:string[])
                n202 = Match First String(2:w326, 3:w331) -> (0:w327:i32)  [unwired: 1 out]
                n203 = property on="Test Ring" class="Ring (strict)"("Value"=w327, "Strings []"=w326) -> ()  [unwired: 2 in, 2 out]
                n204 = property on="Test Ring" class="Ring (strict)"("Visible"=TRUE) -> ()  [unwired: 2 in, 2 out]
                n205 = property on="Test Slider" class="Slide (strict)"("Visible"=FALSE) -> ()  [unwired: 2 in, 2 out]
              }
              frame "Color Enable  **" {
                n206 = Index Array(array=w338, index=4) -> (element=w339:cluster{string[]})
                n207 = call <vilib>:"NT Read String.vi"("Name"=w341) -> ("String"=w340:string)  [unwired: 9 in, 1 out]
                n208 = Unbundle(w339) -> (w335:string[])
                n209 = Match First String(2:w335, 3:w340) -> (0:w336:i32)  [unwired: 1 out]
                n210 = property on="Test Ring" class="Ring (strict)"("Value"=w336, "Strings []"=w335) -> ()  [unwired: 2 in, 2 out]
                n211 = property on="Test Ring" class="Ring (strict)"("Visible"=TRUE) -> ()  [unwired: 2 in, 2 out]
                n212 = property on="Test Slider" class="Slide (strict)"("Visible"=FALSE) -> ()  [unwired: 2 in, 2 out]
              }
              frame Default {
                n213 = property on="Test Ring" class="Ring (strict)"("Visible"=FALSE) -> ()  [unwired: 2 in, 2 out]
                n214 = property on="Test Slider" class="Slide (strict)"("Visible"=FALSE) -> ()  [unwired: 2 in, 2 out]
              }
              frame "Brightness  **", "Color Level  **", "Compression  **", "FPS  **", "Sharpness  **" {
                n215 = call <vilib>:"NT Read Number.vi"("Name"=w347) -> ("Numeric"=w346:dbl)  [unwired: 9 in, 1 out]
                n216 = local write "Test Slider"(w346) -> ()
                n217 = property on="Test Slider" class="Slide (strict)"("Visible"=TRUE, "Scale.Maximum"=100.0 ("Scale.Range:Maximum")) -> ()  [unwired: 2 in, 2 out]
                n218 = property on="Test Ring" class="Ring (strict)"("Visible"=FALSE) -> ()  [unwired: 2 in, 2 out]
              }
            }
          }
        }
        n219 = property on="Progress" class="Clust (strict)"("Visible"=FALSE) -> ()  [unwired: 2 in, 2 out]
      }
      event "Test Name": Mouse Enter {
        # "Populate the ring with the list of tests"
        n220 = event-data() -> ()  [unwired: 1 in, 1 out]
        n221 = call <vilib>:"NT Read String Array.vi"("Name"="TestMode/TestList") -> ("String Array"=w355:string[])  [unwired: 9 in, 1 out]
        n222 = Build Array (concatenate)("Select the test to run...", w355) -> (w354:string[])
        n223 = property on="Test Name" class="Ring (strict)"("Strings []"=w354) -> ()  [unwired: 2 in, 2 out]
      }
      event "Test Name": Value Change {
        w357 = FALSE ("Visible")
        # "Tell the robot the test name to run"
        n224 = event-data() -> ("NewVal"=w361:u16)  [unwired: 1 in]
        n225 = property on="Test Name" class="Ring (strict)"() -> ("Strings []"=w362:string[])  [unwired: 2 in, 2 out]
        n226 = local write "Progress"(T8 {"Test Progress"=0, "Test Progress Text"=""} ("Progress")) -> ()
        n227 = Index Array(array=w362, index=w361) -> (element=w360:string)
        n228 = call <vilib>:"NT Write String.vi"("String"=w360, "Name"="TestMode/TestName") -> ()  [unwired: 9 in, 1 out]
        n229 = property on="Progress" class="Clust (strict)"("Visible"=TRUE) -> ()  [unwired: 2 in, 2 out]
        n230 = property on="Motor" class="Clust (strict)"("Visible"=w357) -> ()  [unwired: 2 in, 2 out]
        n231 = property on="Test Slider" class="Slide (strict)"("Visible"=w357) -> ()  [unwired: 2 in, 2 out]
        n232 = property on="On/Off" class="Bool (strict)"("Visible"=w357) -> ()  [unwired: 2 in, 2 out]
        n233 = property on="Rev/Fwd" class="Clust (strict)"("Visible"=w357) -> ()  [unwired: 2 in, 2 out]
        n234 = property on="Test Ring" class="Ring (strict)"("Visible"=w357) -> ()  [unwired: 2 in, 2 out]
      }
      event "Select Auto": Mouse Enter {
        # "Populate the combo box with the list of autonomous options"
        n235 = event-data() -> ()  [unwired: 1 in, 1 out]
        n236 = call <vilib>:"NT Read String Array.vi"("Name"="Auto List") -> ("String Array"=w364:string[])  [unwired: 9 in, 1 out]
        n237 = property on="Select Auto" class="CmbBox"("Strings[]"=w364) -> ()  [unwired: 2 in, 2 out]
      }
      event "Select Auto": Value Change {
        # "User modified the Auto Selection. Write to NT variable so robot knows."
        n238 = event-data() -> ("NewVal"=w367:string)  [unwired: 1 in]
        n239 = call <vilib>:"NT Write String.vi"("String"=w367, "Name"="Auto Selector") -> ()  [unwired: 9 in, 1 out]
      }
      event "Command Selection": Value Change {
        # "Get the params and show in table"
        n240 = event-data() -> ("NewVal"=w373:i32)  [unwired: 1 in]
        n241 = property on="Command Selection" class="MCListbox (strict)"() -> ("ItemNames"=w371:string[][])  [unwired: 2 in, 2 out]
        n242 = call <vilib>:"WPI_DashboardUpdate Command Params.vi"("NewVal"=w373, "Commands"=w371, "Param Tbl"=w372) -> ()  [unwired: 8 in, 1 out]
      }
      event "Execute Command": Value Change {
        # "Started one, Unique ID holds\nresponse"
        n243 = event-data() -> ()  [unwired: 1 in, 1 out]
        n244 = property on="Command Selection" class="MCListbox (strict)"() -> ("ItemNames"=w384:string[][])  [unwired: 2 in, 2 out]
        n245 = Index Array(array=w384, index (row)="Command Selection", index (col)=0) -> (element=w382:string)
        n246 = call <vilib>:"Invoke Commands.vi"("Command Params"="Command Params", "Function Name"=w382) -> ("Params"=w378:u8, "Started"=w377:bool)  [unwired: 7 in, 1 out]
        n247 = Array Subset(array="Command Params", length (row)=w378) -> (w379:string[][])  [unwired: 3 in]
        n248 = Select(t="Executing" ("Cmd Status"), s=w377, f="" ("Cmd Status")) -> (s? t:f=→"Cmd Status":string)
      }
      event "Command Selection": Double Click {
        n249 = event-data() -> ("Row"=w392:i32)  [unwired: 1 in]
        n250 = property on="Command Selection" class="MCListbox (strict)"() -> ("ItemNames"=w395:string[][])  [unwired: 2 in, 2 out]
        n251 = local read "Command Params"() -> (w391:string[][])
        n252 = Index Array(array=w395, index (row)=w392, index (col)=0) -> (element=w393:string)
        n253 = call <vilib>:"Invoke Commands.vi"("Command Params"=w391, "Function Name"=w393) -> ("Params"=w390:u8, "Started"=w385:bool)  [unwired: 7 in, 1 out]
        n254 = Array Subset(array=w391, length (row)=w390) -> (w389:string[][])  [unwired: 3 in]
        n255 = Select(t="Executing" ("Cmd Status"), s=w385, f="" ("Cmd Status")) -> (s? t:f=w386:string)
        n256 = local write "Cmd Status"(w386) -> ()
      }
      event "CheckList": Double Click {
        # "Shift clears all"
        # "Update symbols on the listbox"
        n257 = event-data() -> ("PlatMods.Shift"=w397:bool, "Row"=w399:i32)  [unwired: 1 in]
        n258 = case shown="True" w397 {
          tunnel: w399 -> [w403 _]
          tunnel: 1 -> [w402 _]
          frame False {
            n259 = property on="CheckList" class="LstBox (strict)"() -> ("Item Symbols"=w401:i32[])  [unwired: 2 in, 2 out]
            n260 = Replace Array Subset(array=w401, new element=w402, index=w403) -> (w400:i32[])
            n261 = property on="CheckList" class="LstBox (strict)"("Item Symbols"=w400) -> ()  [unwired: 2 in, 2 out]
          }
          frame True {
            w404 = 0 ("Top Row")
            n262 = property on="CheckList" class="LstBox (strict)"() -> ("Number of Rows"=w406:u32)  [unwired: 2 in, 2 out]
            n263 = Initialize Array(0, w406) -> (w405:i32[])
            n264 = property on="CheckList" class="LstBox (strict)"("Top Row"=w404, "Value"=w404, "Item Symbols"=w405) -> ()  [unwired: 2 in, 2 out]
          }
        }
      }
      event "CheckList": Key Down {
        # "Update symbols on the listbox\nLeft and right keys check and uncheck"
        n265 = event-data() -> ("VKey"=w410:T22)  [unwired: 1 in]
        n266 = case shown="\"Left\", \"Right\"" w410 {
          selector: w410 -> [w415 _]
          tunnel: eventvkey."Left" ("VKey") -> [w413 _]
          frame "Left", "Right" {
            n267 = Equal?(x=w413, y=w415) -> (x = y?=w414:bool)
            n268 = Select(t=0, s=w414, f=1) -> (s? t:f=w416:i32)
            n269 = property on="CheckList" class="LstBox (strict)"() -> ("Item Symbols"=w419:i32[])  [unwired: 2 in, 2 out]
            n270 = Replace Array Subset(array=w419, new element=w416, index="CheckList") -> (w418:i32[])
            n271 = property on="CheckList" class="LstBox (strict)"("Item Symbols"=w418) -> ()  [unwired: 2 in, 2 out]
          }
          frame Default {
          }
        }
      }
      event "Motor.Enable": Value Change {
        # "When the test mode otor enable helper is set, update that\ntree row item's value"
        n272 = event-data() -> ("NewVal"=w425:bool)  [unwired: 1 in]
        n273 = Unbundle("Motor") -> ("Value"=w424:dbl)  [unwired: 1 out]
        n274 = Select(t=w424, s=w425, f=0.0) -> (s? t:f=w422:dbl)
        n275 = call <vilib>:"NT Write Number.vi"("Numeric"=w422, "Name"=w421) -> ()  [unwired: 9 in, 1 out]
      }
      event "Test Slider": Value Change {
        # "When the test mode slider helper is set, update that\ntree row item's value"
        n276 = event-data() -> ("NewVal"=w428:dbl)  [unwired: 1 in]
        n277 = call <vilib>:"NT Write Number.vi"("Numeric"=w428, "Name"=w429) -> ()  [unwired: 9 in, 1 out]
      }
      event "On/Off": Value Change {
        # "When the test mode on/off helper value is set, update that\ntree row item's value"
        n278 = event-data() -> ("NewVal"=w433:bool)  [unwired: 1 in]
        n279 = Boolean To (0,1)(Boolean=w433) -> (0, 1=w432:i16)
        n280 = call <vilib>:"NT Write Number.vi"("Numeric"=w432, "Name"=w431) -> ()  [unwired: 9 in, 1 out]
      }
      event "Rev/Fwd": Value Change {
        # "When the test mode helper value for relays is set, update that\ntree row item's value"
        n281 = event-data() -> ("NewVal.Forward"=w441:bool, "NewVal.Reverse"=w440:bool)  [unwired: 1 in]
        n282 = Boolean To (0,1)(Boolean=w441) -> (0, 1=w437:i16)
        n283 = Boolean To (0,1)(Boolean=w440) -> (0, 1=w439:i16)
        n284 = Negate(x=w439) -> (-x=w438:i16)
        n285 = Add(x=w437, y=w438) -> (x+y=w436:i16)
        n286 = call <vilib>:"NT Write Number.vi"("Numeric"=w436, "Name"=w435) -> ()  [unwired: 9 in, 1 out]
      }
      event "Test Ring": Value Change {
        # "When a test mode helper value is selected from the ring,\nset the tree item's variable to the string value"
        n287 = event-data() -> ("NewVal"=w445:u16)  [unwired: 1 in]
        n288 = property on="Test Ring" class="Ring (strict)"() -> ("Strings []"=w446:string[])  [unwired: 2 in, 2 out]
        n289 = Index Array(array=w446, index=w445) -> (element=w444:string)
        n290 = call <vilib>:"NT Write String.vi"("String"=w444, "Name"=w443) -> ()  [unwired: 9 in, 1 out]
      }
      event "Rec Mode": Value Change {
        # "Update globals for recording mode and path to read log from.\nClear when logging and let NetworkTables set path for vision to\nuse."
        n291 = event-data() -> ("NewVal"=w457:enum32{"Stop", "Record", "Playback"})  [unwired: 1 in]
        n292 = global write "WPI_DashboardLogging Global.vi" "Logging Filename"(path "") -> ()
        n293 = global write "WPI_DashboardLogging Global.vi" "Recording"(w457) -> ()
        n294 = case shown="\"Playback\"" w457 {
          tunnel: w456 -> [_ w459 w468]
          tunnel: [_ _ w467] -> w454
          tunnel: [_ _ w466] -> _
          tunnel: w452 -> [_ _ w464]
          tunnel: cluster{i32, i32} {-250, 170} -> [_ _ w463]
          tunnel: [_ _ T23 {"Image Size"=TRUE, "Image Type"=TRUE, "Pixel Value"=TRUE, "ROI Information"=TRUE, "Zoom Factor"=FALSE} ("Image Information Shown:All Elements")] -> w447
          tunnel: [_ _ TRUE ("Zoom Factor")] -> w448
          tunnel: w450 -> [_ _ w460]
          frame Default {
          }
          frame "Stop", "Record" {
            # "Place Window too"
            n295 = invoke class="VI" method="FP.Close"(reference=w459) -> (reference out=w458:refnum<vi>)  [unwired: 2 in, 2 out]
            n296 = invoke class="VI" method="Abort VI"(reference=w458) -> ()  [unwired: 2 in, 3 out]
          }
          frame "Playback" {
            n297 = call "Open Playback Panel.vi"("Offset"=w463, "DB VI Ref"=w464, "Playback in"=w468) -> ("Playback out"=w465:refnum<vi>)  [unwired: 8 in]
            n298 = register-events(w465, w460) -> (reference out=w467:refnum<event-registration>, error out=w466:errorcluster)  [unwired: 2 in]
          }
        }
        n299 = property on="Camera Image Right" class="ImageControl"("Image Information Shown"=w447, "Image Information Visible"=w448) -> ()  [unwired: 2 in, 2 out]
        n300 = property on="Camera Image" class="ImageControl"("Image Information Shown"=w447, "Image Information Visible"=w448) -> ()  [unwired: 2 in, 2 out]
        n301 = call <vilib>:"WPI_DashboardNT Log FieldName Cache.vi"("Operation"=enum16{"Lookup/Add", "Index", "Clear"}."Clear") -> ()  [unwired: 8 in, 3 out]
      }
      event Panel Close {
        w470 = enum32{"Stop", "Record", "Playback"}."Stop" ("Rec Mode")
        # "Playback window has been closed, abort"
        n302 = event-data() -> ()  [unwired: 1 in, 4 out]
        n303 = local write "Rec Mode"(w470) -> ()
        n304 = global write "WPI_DashboardLogging Global.vi" "Recording"(w470) -> ()
      }
      event Panel Close {
        # "Abort playback window and ourself"
        n305 = event-data() -> ()  [unwired: 1 in, 4 out]
        n306 = invoke class="VI" method="FP.Close"(reference=w474) -> (reference out=w473:refnum<vi>)  [unwired: 2 in, 2 out]
        n307 = invoke class="VI" method="Abort VI"(reference=w473) -> (error out=w472:errorcluster)  [unwired: 2 in, 2 out]
        n308 = invoke class="VI" method="Abort VI"(error in=w472) -> ()  [unwired: 2 in, 3 out]
      }
      event User Event {
        n309 = event-data() -> ("IDs"=w481:cluster{"RPC field ID":u16, "Unique ID":u16}, "String"=w480:string)  [unwired: 1 in]
        n310 = Bundle("IDs"=w481, "String"=w480) -> (w479:T12)  [unwired: 1 in]
        n311 = call <vilib>:"Retrieve RPC Response.vi"("RPC Response"=w479) -> ("Output"=w477:string[][])  [unwired: 10 in]
        n312 = Build Array (concatenate)(w475, w477) -> (w476:string[][])
        n313 = local write "Command Params"(w476) -> ()
        n314 = local write "Cmd Status"("" ("Cmd Status")) -> ()
      }
      event "Tree": Double Click {
        n315 = event-data() -> ("PlatMods"=w487:T26, "Tag"=w484:string)  [unwired: 1 in]
        n316 = Unbundle(w487) -> ("Shift"=w486:bool)  [unwired: 4 out]
        n317 = String Subset(string=w484, length (rest)=1 ("length (rest)")) -> (substring=w483:string)  [unwired: 1 in]
        n318 = Not(x=w486) -> (.not. x?=w485:bool)
        n319 = case shown="\"/\"" w483 {
          tunnel: w484 -> [_ w490]
          tunnel: w485 -> [_ w489]
          frame Default {
          }
          frame "/" {
            n320 = call <vilib>:"NT Update Persistence.vi"("Persistence"=w489, "Name"=w490) -> ()  [unwired: 9 in, 1 out]
          }
        }
      }
    }
  }
  n321 = while {
    tunnel: w65 -> [w492]
    i -> [w495]
    stop <- FALSE stop-if-true
    n322 = Wait (ms)(milliseconds to wait=u32 100) -> ()  [unwired: 1 out]
    n323 = case shown="\"Playback\"" "Rec Mode" {
      tunnel: w495 -> [_ _ w510]
      tunnel: [u32 2829099 ("Base Color") u32 11141120 ("Target Color") w499] -> w491
      frame "Stop", Default {
        # "Reset the color, extra updates don't cost much"
      }
      frame "Record" {
      }
      frame "Playback" {
        # "Playback"
        n324 = Quotient & Remainder(x=w510, y=u32 50 ("milliseconds to wait")) -> (x-y*floor(x/y)=w506:u32)  [unwired: 1 out]
        n325 = Divide(x=w506, y=u32 50 ("milliseconds to wait")) -> (x/y=w503:dbl)
        n326 = Multiply(x=6.283185307179586, y=w503) -> (x*y=w508:dbl)
        n327 = Sine(x=w508) -> (sin(x)=w507:dbl)
        n328 = Absolute Value(x=w507) -> (abs(x)=w500:dbl)
        n329 = call "Interpolate RGB Color.vi"("Proportion"=w500, "Target Color"=u32 30976, "Base Color"=u32 2829099) -> ("Result Color"=w499:u32)  [unwired: 8 in]
      }
    }
    n330 = property class="Pane"(reference=w492, "PaneColor"=w491) -> ()  [unwired: 1 in, 2 out]
  }
  n331 = local write "Dashboard Tab"(T2."Drive" ("Dashboard Tab")) -> ()
  n332 = property on="On/Off" class="Bool (strict)"("Visible"=w41) -> ()  [unwired: 2 in, 2 out]
  n333 = property on="Motor" class="Clust (strict)"("Visible"=w41) -> ()  [unwired: 2 in, 2 out]
  n334 = property on="Progress" class="Clust (strict)"("Visible"=w41) -> ()  [unwired: 2 in, 2 out]
  n335 = property on="Test Ring" class="Ring (strict)"("Visible"=w41) -> ()  [unwired: 2 in, 2 out]
  n336 = property on="Rev/Fwd" class="Clust (strict)"("Visible"=w41) -> ()  [unwired: 2 in, 2 out]
  n337 = while {
    tunnel: u16 1741 ("timeout ms (25000)") -> [w512]
    stop <- FALSE stop-if-true
    n338 = TCP Create Listener(10:w512) -> (0:w511:errorcluster, 3:w513:refnum<k5>)  [unwired: 4 in, 1 out]
    n339 = case shown="No Error" w511 {
      selector: w511 -> [w515 _]
      tunnel: w513 -> [w516 _]
      frame No Error {
        n340 = while {
          tunnel: w516 -> [w519]
          tunnel: w515 -> [w518]
          stop <- FALSE stop-if-true
          n341 = TCP Wait On Listener(8:w518, 11:w519) -> (0:w520:errorcluster, 4:w521:refnum<k5>)  [unwired: 2 in, 3 out]
          n342 = local write "TCP"(w521) -> ()
          n343 = case shown="No Error" w520 {
            frame No Error {
            }
            frame Error {
              n344 = Wait (ms)(milliseconds to wait=u32 1000) -> ()  [unwired: 1 out]
            }
          }
        }
      }
      frame Error {
        n345 = Wait (ms)(milliseconds to wait=u32 1000) -> ()  [unwired: 1 out]
      }
    }
  }
  n346 = local write "Command Selection"(u16 0 ("milliseconds to wait")) -> ()
  n347 = local write "Command Params"(string[][] [] ("Command Params")) -> ()
  n348 = global write "WPI_DashboardLogging Global.vi" "Recording"(w59) -> ()
  n349 = local write "Rec Mode"(w59) -> ()
  n350 = call <vilib>:"NT Write String.vi"("String"="Select Auto", "Name"="Auto Selector") -> ()  [unwired: 9 in, 1 out]
